vi "Helicopter Read-Write.vi"(0 "Hellicopter Tasks Input":T2, 2 "Pitch Calib":T1={"Array"=[[80.0, 1.0, 1.0, 1.0, 1.0, 1.0, 1.0, 1.0, 1.0], [70.0, 0.875, 0.0, 0.0, 0.0, 0.0, 0.0, 0.0, 0.0], [60.0, 0.75, 0.0, 0.0, 0.0, 0.0, 0.0, 0.0, 0.0], [50.0, 0.625, 0.0, 0.0, 0.0, 0.0, 0.0, 0.0, 0.0], [40.0, 0.5, 0.0, 0.0, 0.0, 0.0, 0.0, 0.0, 0.0], [30.0, 0.375, 0.0, 0.0, 0.0, 0.0, 0.0, 0.0, 0.0], [20.0, 0.25, 0.0, 0.0, 0.0, 0.0, 0.0, 0.0, 0.0], [10.0, 0.125, 0.0, 0.0, 0.0, 0.0, 0.0, 0.0, 0.0], [0.0, 0.0, 0.0, 0.0, 0.0, 0.0, 0.0, 0.0, 0.0], [-10.0, -0.125, 0.0, 0.0, 0.0, 0.0, 0.0, 0.0, 0.0], [-20.0, -0.25, 0.0, 0.0, 0.0, 0.0, 0.0, 0.0, 0.0], [-30.0, -0.375, 0.0, 0.0, 0.0, 0.0, 0.0, 0.0, 0.0], [-40.0, -0.5, 0.0, 0.0, 0.0, 0.0, 0.0, 0.0, 0.0], [-50.0, -0.625, 0.0, 0.0, 0.0, 0.0, 0.0, 0.0, 0.0], [-60.0, -0.75, 0.0, 0.0, 0.0, 0.0, 0.0, 0.0, 0.0], [-70.0, -0.875, 0.0, 0.0, 0.0, 0.0, 0.0, 0.0, 0.0], [-80.0, -1.0, 0.0, 0.0, 0.0, 0.0, 0.0, 0.0, 0.0]], "Operation"=FALSE}, 7 "Fan Input":dbl[](array[numeric]) format="%0.2f", 11 "Error In":errorcluster) -> (4 "Hellicopter Tasks Output":T2, 6 "Elevation":dbl format="%0.2f", 8 "Pitch":dbl format="%0.2f", 10 "Travel":dbl format="%0.2f", 15 "Error Out":errorcluster)   [LabVIEW 2017]
uses:
  Pitch Array 1.ctl
  <vilib>/DAQmx/read.llb/DAQmx Read (Analog 2D DBL NChan NSamp).vi
  <vilib>/DAQmx/read.llb/DAQmx Read (Counter DBL 1Chan 1Samp).vi
  <vilib>/Analysis/baseanly.llb/Mean (DBL).vi
  <vilib>/DAQmx/write.llb/DAQmx Write (Analog 1D DBL NChan 1Samp).vi
  <vilib>/DAQmx/write.llb/DAQmx Write (Digital 1D Bool NChan 1Samp 1Line).vi
  <vilib>/DAQmx/miscellaneous.llb/DAQmx Fill In Error Info.vi
  <vilib>/Analysis/NI_AALBase.lvlib
panel:
  # "Calibration\nMode"
  # "Operating\nMode"
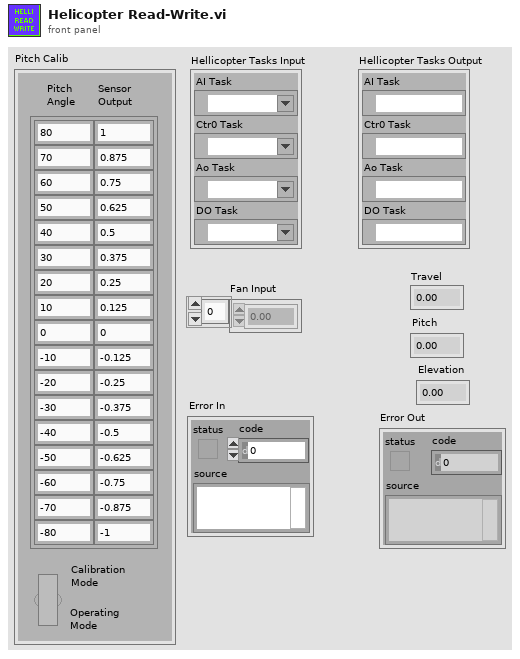
[diagram p1: front panel]
types:
  T1 = typedef "Pitch Array 1.ctl" = cluster{"Array":dbl[][], "Operation":bool}
  T2 = cluster{"AI Task":refnum<k21>, "Ctr0 Task":refnum<k21>, "Ao Task":refnum<k21>, "DO Task":refnum<k21>}
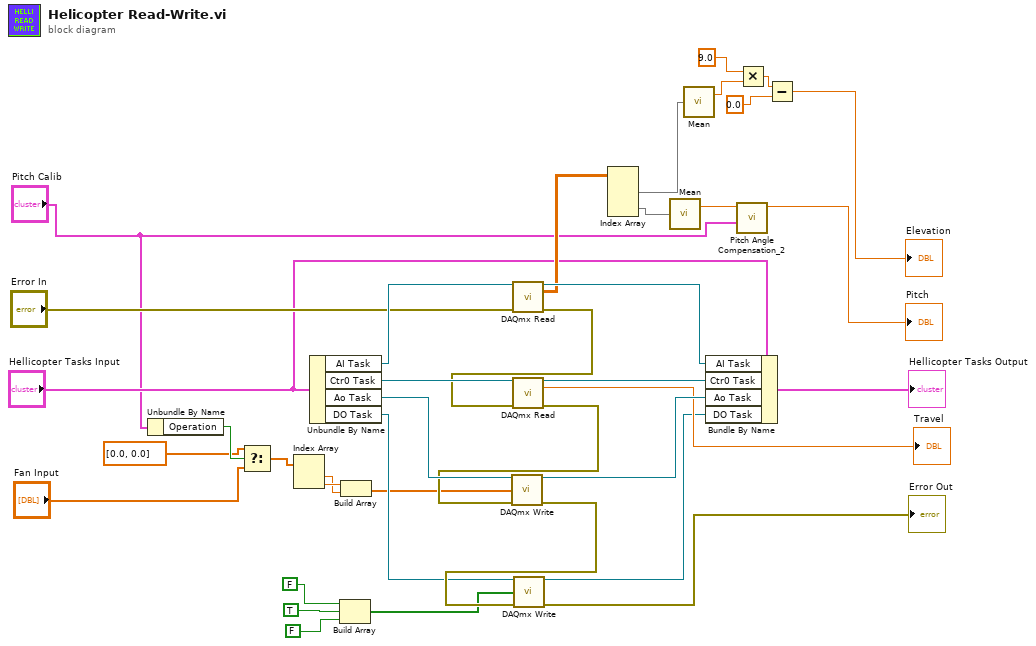
[diagram p0: block diagram]
diagram:
  n1 = Unbundle By Name("Pitch Calib") -> ("Operation"=w4:bool)
  n2 = Select(t=dbl[] [0.0, 0.0] ("f"), s=w4, f="Fan Input") -> (s? t:f=w6:dbl[])
  n3 = Index Array(array=w6) -> (element #1=w7:dbl, element #2=w8:dbl)  [unwired: 2 in]
  n4 = Unbundle By Name("Hellicopter Tasks Input") -> ("AI Task"=w35:refnum<k21>, "Ctr0 Task"=w33:refnum<k21>, "Ao Task"=w34:refnum<k21>, "DO Task"=w16:refnum<k21>)
  n5 = Build Array(FALSE, TRUE ("element"), FALSE ("element")) -> (w14:bool[])
  n6 = Build Array(w8, w7) -> (w9:dbl[])
  n7 = call-poly <vilib>:"DAQmx Read.vi"("task/channels in"=w35, "error in"="Error In") -> ("task out"=w38:refnum<k21>, "data"=w21:dbl[][], "error out"=w32:errorcluster)  [unwired: 11 in]
  n8 = call-poly <vilib>:"DAQmx Read.vi"("task/channels in"=w33, "error in"=w32) -> ("task out"=w37:refnum<k21>, "data"=→"Travel":dbl, "error out"=w31:errorcluster)  [unwired: 11 in]
  n9 = call-poly <vilib>:"DAQmx Write.vi"("task/channels in"=w34, "data"=w9, "error in"=w31) -> ("task out"=w36:refnum<k21>, "error out"=w20:errorcluster)  [unwired: 10 in, 1 out]
  n10 = call-poly <vilib>:"DAQmx Write.vi"("task/channels in"=w16, "data"=w14, "error in"=w20) -> ("task out"=w15:refnum<k21>, "error out"=→"Error Out":errorcluster)  [unwired: 10 in, 1 out]
  n11 = Index Array(array=w21) -> (element #1=w23:dbl[], element #2=w22:dbl[])  [unwired: 4 in]
  n12 = call-poly <vilib>:"Mean.vi"("X"=w22) -> ("mean"=w10:dbl)  [unwired: 1 out]
  n13 = call-poly <vilib>:"Mean.vi"("X"=w23) -> ("mean"=w28:dbl)  [unwired: 1 out]
  n14 = Bundle By Name(cluster="Hellicopter Tasks Input", "AI Task"=w38, "Ctr0 Task"=w37, "Ao Task"=w36, "DO Task"=w15) -> (→"Hellicopter Tasks Output":T2)
  n15 = call "Pitch Angle Compensation_2.vi"("Pitch Calib"="Pitch Calib", "Sensor Input"=w10) -> ("Pitch Angle"=→"Pitch":dbl)  [unwired: 9 in]
  n16 = Multiply(x=9.0, y=w28) -> (x*y=w25:dbl)
  n17 = Subtract(x=w25, y=0.0) -> (x-y=→"Elevation":dbl)
